vi "温度补偿.vi"() -> ()   [LabVIEW 2016, in "斯坦道CODMn.lvlib"]
uses:
  <vilib>/Analysis/6fits.llb/Curve Fitting Criteria.ctl
  <vilib>/Plasmionique/MB Master/MB Master.lvlib
  <vilib>/Analysis/NI_AALPro.lvlib
panel:
  in  "读取":bool
  in  "写入":bool
  in  "关闭":bool
  in  "曲线模型":T1 {"二次方程"."x^2" format="%#.6g"; "二次方程"."K" format="%#.6g"; "二次方程"."B" format="%#.6g"; "r^2" format="%.7f"; "测量吸光度5" format="%#.6f"; "测量吸光度4" format="%#.6f"; "测量吸光度3" format="%#.6f"; "测量吸光度2" format="%#.6f"; "测量吸光度1" format="%#.6f"}
  # "温度"
  # "滴定数"
  # "温度一"
  # "温度二"
  # "温度三"
  # "温度四"
  # "温度五"
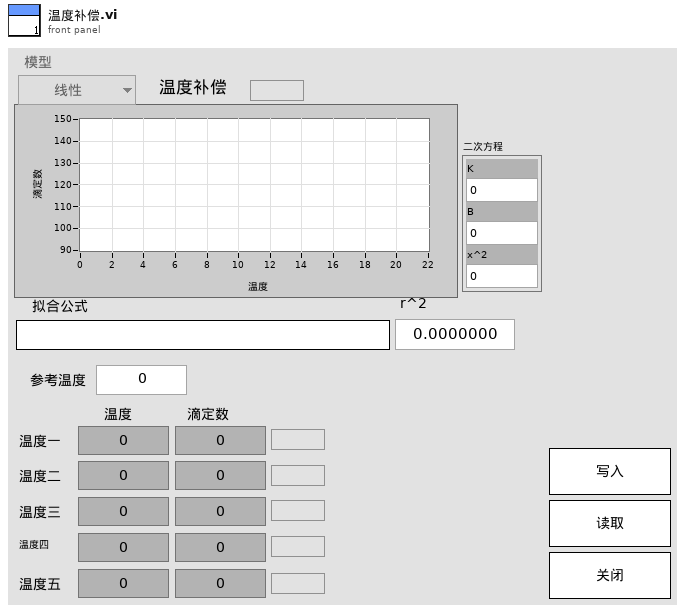
[diagram p1: front panel]
types:
  T1 = cluster{"标液浓度1":dbl, "测量吸光度1":dbl, "样品1启用":bool, "标液浓度2":dbl, "测量吸光度2":dbl, "样品2启用":bool, "标液浓度3":dbl, "测量吸光度3":dbl, "样品3启用":bool, "标液浓度4":dbl, "测量吸光度4":dbl, "样品4启用":bool, "标液浓度5":dbl, "测量吸光度5":dbl, "样品5启用":bool, "模型":enum32{"线性", "多项式", "折线"}, "XY图":cluster{"X Values":dbl[], "Y Values":dbl[]}[], "拟合公式":string, "r^2":dbl, "二次方程":cluster{"K":dbl, "B":dbl, "x^2":dbl}, "参考温度":dbl, "温度补偿":bool}
  T2 = typedef "NI_AALPro.lvlib/Curve Fitting Criteria.ctl" = u16
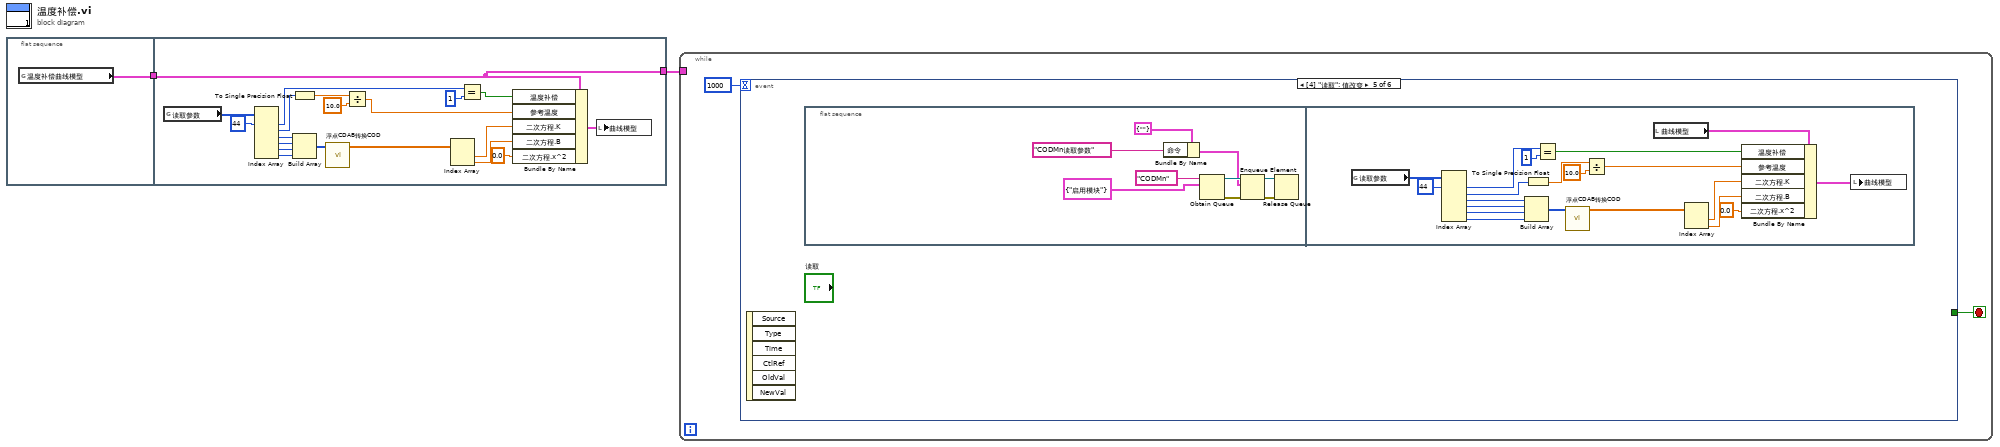
[diagram p0: block diagram]
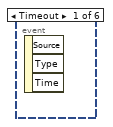
[diagram p2: hidden frame]
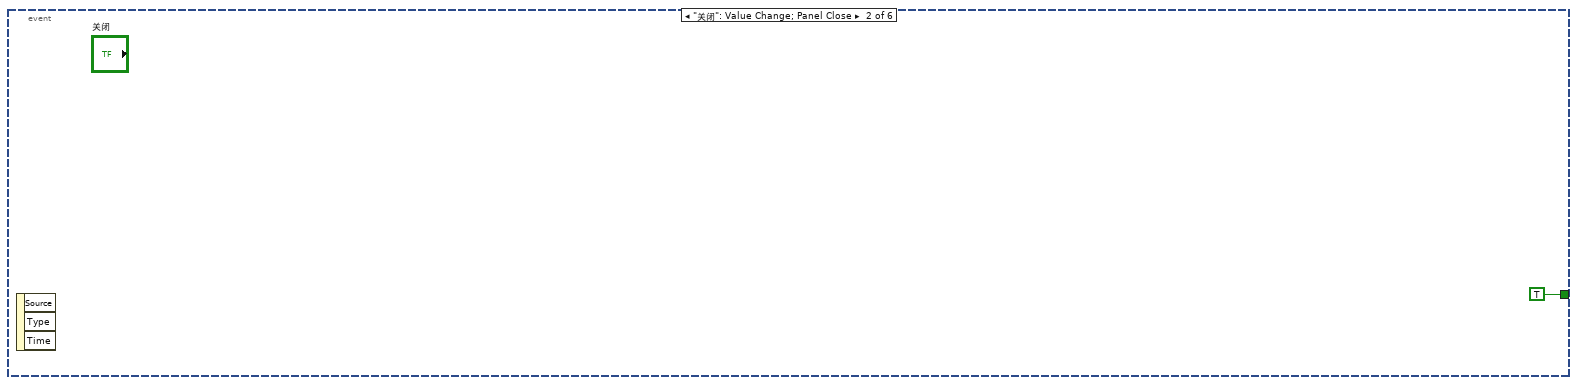
[diagram p3: hidden frame]
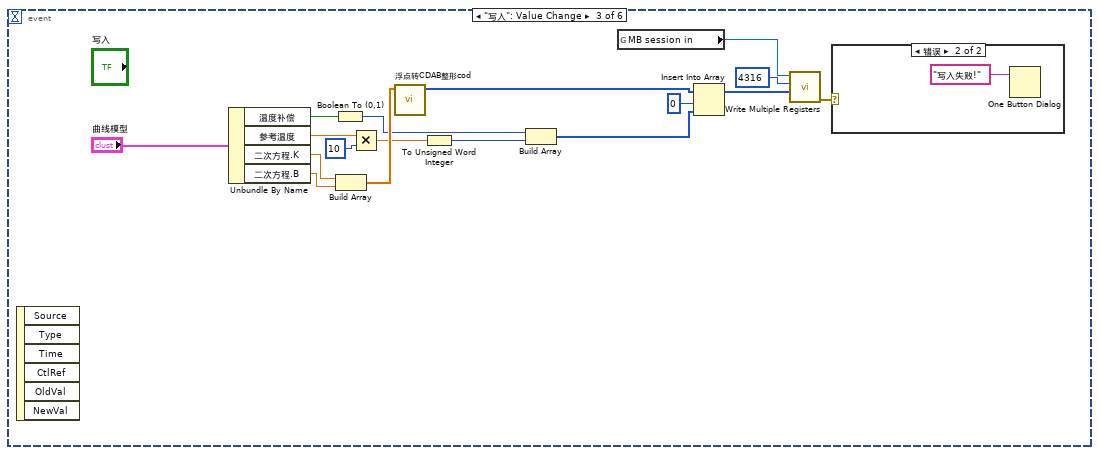
[diagram p4: hidden frame]
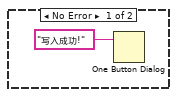
[diagram p5: hidden frame]
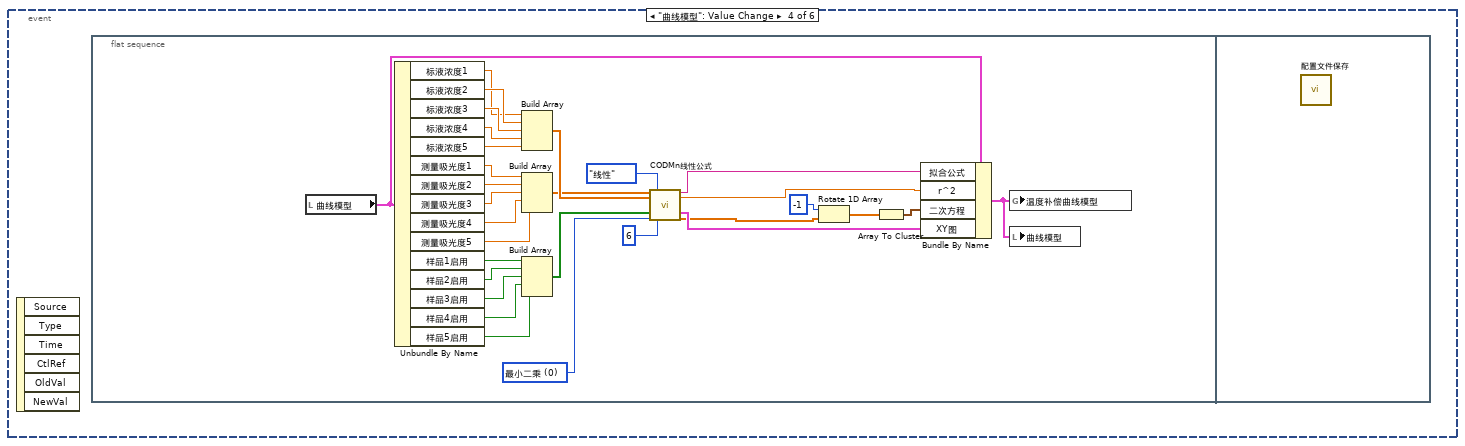
[diagram p6: hidden frame]
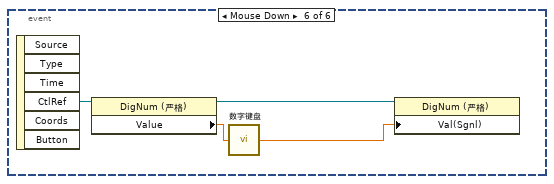
[diagram p7: hidden frame]
diagram:
  n1 = flat-sequence {
    tunnel: [w3] -> w1
    tunnel: [w21] -> w2
    tunnel: w1 -> [w21]
    frame #0 {
      n2 = global read "CODMn断电保存全局变量.vi" "温度补偿曲线模型"() -> (w3:T1)
    }
    frame #1 {
      n3 = global read "COD内部交互全局.vi" "读取参数"() -> (w23:u16[])
      n4 = Index Array(array=w23, index #1=44 ("索引")) -> (element #1=w8:u16, element #2=w5:u16, element #3=w18:u16, element #4=w17:u16, element #5=w16:u16, element #6=w15:u16)  [unwired: 5 in]
      n5 = To Single Precision Float(number=w5) -> (single precision float=w4:sgl)
      n6 = Build Array(w18, w17, w16, w15) -> (w14:u16[])
      n7 = call "浮点CDAB转换COD.vi"("数组"=w14) -> ("数组 2"=w13:sgl[])  [unwired: 10 in]
      n8 = Divide(x=w4, y=sgl 10.0) -> (x/y=w19:sgl)
      n9 = Index Array(array=w13) -> (element #1=w12:sgl, element #2=w11:sgl)  [unwired: 2 in]
      n10 = Equal?(x=w8, y=u16 1) -> (x = y?=w6:bool)
      n11 = Bundle By Name(cluster=w21, "温度补偿"=w6, "参考温度"=w19, "二次方程.K"=w12, "二次方程.B"=w11, "二次方程.x^2"=0.0) -> (w20:T1)
      n12 = local write "曲线模型"(w20) -> ()
    }
  }
  n13 = while {
    tunnel: w2 -> [_]
    stop <- w25 stop-if-true
    n14 = event shown="[4] \"读取\": 值改变" {
      selector: _ -> [_ _ _ _ _ _]
      dyn-events: _ -> [_ _ _ _ _ _]
      timeout: 1000 -> [_ _ _ _ _ _]
      tunnel: [_ TRUE _ _ _ _] -> w25
      event Timeout {
        n15 = event-data() -> ()  [unwired: 1 in, 3 out]
      }
      event "关闭": Value Change; Panel Close {
        n16 = event-data() -> ()  [unwired: 1 in, 3 out]
      }
      event "写入": Value Change {
        n17 = event-data() -> ()  [unwired: 1 in, 6 out]
        n18 = Unbundle By Name("曲线模型") -> ("温度补偿"=w29:bool, "参考温度"=w35:dbl, "二次方程.K"=w40:dbl, "二次方程.B"=w39:dbl)
        n19 = Boolean To (0,1)(Boolean=w29) -> (0, 1=w28:i16)
        n20 = Build Array(w40, w39) -> (w38:dbl[])
        n21 = Multiply(x=w35, y=u16 10 ("新元素/子数组")) -> (x*y=w33:dbl)
        n22 = call "浮点转CDAB整形cod.vi"("浮点数"=w38) -> ("CDAB整形输出"=w37:u16[])  [unwired: 10 in]
        n23 = To Unsigned Word Integer(number=w33) -> (unsigned 16bit integer=w30:u16)
        n24 = Build Array(w28, w30) -> (w27:u16[])
        n25 = global read "COD浓度全局变量.vi" "MB session in"() -> (w42:refnum<class "MB_Master.lvclass">)
        n26 = Insert Into Array(array=w37, index=0 ("索引"), new element=w27) -> (w32:u16[])
        n27 = call <vilib>:"Write Multiple Registers.vi"("values"=w32, "starting address"=u16 4316, "MB session in"=w42) -> ("error out"=w31:errorcluster)  [unwired: 7 in, 1 out]
        n28 = case shown="错误" w31 {
          frame No Error {
            n29 = One Button Dialog(message="写入成功!" ("消息")) -> ()  [unwired: 1 in, 1 out]
          }
          frame Error {
            n30 = One Button Dialog(message="写入失败!" ("消息")) -> ()  [unwired: 1 in, 1 out]
          }
        }
      }
      event "曲线模型": Value Change {
        n31 = event-data() -> ()  [unwired: 1 in, 6 out]
        n32 = flat-sequence {
          frame #0 {
            w47 = T2 0 items=["最小二乘", "最小绝对残差", "Bisquare"] ("method")
            n33 = local read "曲线模型"() -> (w68:T1)
            n34 = Unbundle By Name(w68) -> ("标液浓度1"=w50:dbl, "标液浓度2"=w51:dbl, "标液浓度3"=w52:dbl, "标液浓度4"=w53:dbl, "标液浓度5"=w54:dbl, "测量吸光度1"=w55:dbl, "测量吸光度2"=w56:dbl, "测量吸光度3"=w57:dbl, "测量吸光度4"=w58:dbl, "测量吸光度5"=w59:dbl, "样品1启用"=w60:bool, "样品2启用"=w61:bool, "样品3启用"=w62:bool, "样品4启用"=w63:bool, "样品5启用"=w64:bool)
            n35 = Build Array(w50, w51, w52, w53, w54) -> (w67:dbl[])
            n36 = Build Array(w55, w56, w57, w58, w59) -> (w66:dbl[])
            n37 = Build Array(w60, w61, w62, w63, w64) -> (w65:bool[])
            n38 = call "CODMn线性公式.vi"("标液浓度"=w66, "滴定数"=w67, "启用"=w65, "method"=w47, "模型"=enum32{"线性", "多项式", "折线"}."线性", "精度"=6) -> ("拟合方程"=w69:string, "r^2"=w70:dbl, "XY图"=w75:cluster{"X Values":dbl[], "Y Values":dbl[]}[], "Polynomial Coefficients"=w74:dbl[])  [unwired: 7 in, 3 out]
            n39 = Rotate 1D Array(1:w74, 2:-1 ("n")) -> (0:w71:dbl[])
            n40 = Array To Cluster(array=w71) -> (cluster=w73:cluster{"[0]":dbl, "[1]":dbl, "[2]":dbl})
            n41 = Bundle By Name(cluster=w68, "拟合公式"=w69, "r^2"=w70, "二次方程"=w73, "XY图"=w75) -> (w46:T1)
            n42 = global write "CODMn断电保存全局变量.vi" "温度补偿曲线模型"(w46) -> ()
            n43 = local write "曲线模型"(w46) -> ()
          }
          frame #1 {
            n44 = call "配置文件保存.vi"() -> ()  [unwired: 12 in]
          }
        }
      }
      event "读取": Value Change {
        n45 = event-data() -> ()  [unwired: 1 in, 6 out]
        n46 = flat-sequence {
          frame #0 {
            n47 = Bundle By Name(cluster=cluster{"命令":string} {"命令"=""} ("元素"), "命令"="CODMn读取参数" ("名称（未命名）")) -> (w78:cluster{"命令":string})
            n48 = Obtain Queue(name (unnamed)="CODMn", element data type=cluster{"命令":string} {"命令"="启用模块"} ("元素")) -> (queue out=w83:refnum<queue>, error out=w84:errorcluster)  [unwired: 3 in, 1 out]
            n49 = Enqueue Element(queue=w83, element=w78, error in (no error)=w84) -> (queue out=w81:refnum<queue>, error out=w82:errorcluster)  [unwired: 1 in, 1 out]
            n50 = Release Queue(queue=w81, error in (no error)=w82) -> ()  [unwired: 1 in, 3 out]
          }
          frame #1 {
            n51 = global read "COD内部交互全局.vi" "读取参数"() -> (w88:u16[])
            n52 = Index Array(array=w88, index #1=44 ("索引")) -> (element #1=w102:u16, element #2=w86:u16, element #3=w92:u16, element #4=w93:u16, element #5=w94:u16, element #6=w95:u16)  [unwired: 5 in]
            n53 = Build Array(w92, w93, w94, w95) -> (w96:u16[])
            n54 = To Single Precision Float(number=w86) -> (single precision float=w85:sgl)
            n55 = Equal?(x=w102, y=u16 1) -> (x = y?=w104:bool)
            n56 = call "浮点CDAB转换COD.vi"("数组"=w96) -> ("数组 2"=w97:sgl[])  [unwired: 10 in]
            n57 = Divide(x=w85, y=sgl 10.0) -> (x/y=w91:sgl)
            n58 = local read "曲线模型"() -> (w87:T1)
            n59 = Index Array(array=w97) -> (element #1=w98:sgl, element #2=w99:sgl)  [unwired: 2 in]
            n60 = Bundle By Name(cluster=w87, "温度补偿"=w104, "参考温度"=w91, "二次方程.K"=w98, "二次方程.B"=w99, "二次方程.x^2"=0.0) -> (w90:T1)
            n61 = local write "曲线模型"(w90) -> ()
          }
        }
      }
      event "曲线模型.标液浓度1", "曲线模型.测量吸光度1", "曲线模型.标液浓度2", "曲线模型.测量吸光度2", "曲线模型.标液浓度3", "曲线模型.测量吸光度3", "曲线模型.标液浓度4", "曲线模型.测量吸光度4", "曲线模型.标液浓度5", "曲线模型.测量吸光度5", "曲线模型.参考温度": Mouse Down {
        n62 = event-data() -> ("CtlRef"=w108:refnum<vi>)  [unwired: 1 in, 5 out]
        n63 = property class="DigNum (严格)"(reference=w108) -> (reference out=w106:refnum<vi>, "Value"=w107:dbl)  [unwired: 1 in, 1 out]
        n64 = call "数字键盘.vi"("OldNumber"=w107) -> ("NewNumber"=w105:sgl)
        n65 = property class="DigNum (严格)"(reference=w106, "Val(Sgnl)"=w105) -> ()  [unwired: 1 in, 2 out]
      }
    }
  }
